vi "Test2.vi"   [LabVIEW 2017]
uses:
  C:/Users/Fred Guo/Desktop/relay.dll
  relay.dll
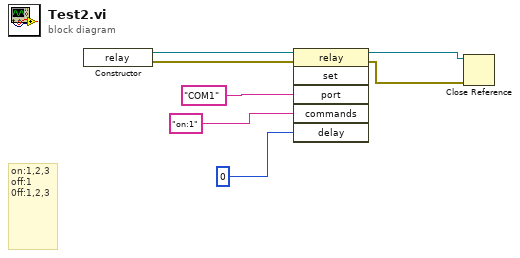
[diagram p0: block diagram]
diagram:
  # "on:1,2,3\noff:1\n0ff:1,2,3"
  n1 = constructor class="relay"() -> (reference out=w7:refnum<k24>, error out=w6:errorcluster)  [unwired: 3 in, 1 out]
  n2 = invoke class="relay" method="set"(reference=w7, error in=w6, "port"="COM1", "commands"="on:1", "delay"=u16 0) -> (reference out=w2:refnum<k24>, error out=w1:errorcluster)  [unwired: 1 in, 4 out]
  n3 = Close Reference(reference=w2, error in (no error)=w1) -> ()  [unwired: 1 out]
